vi "tcpServerSenderLoop.vi"(8 "error in (no error)":errorcluster, 10 "notifier in":refnum<notifier>, 11 "TcpServer in":refnum<class "TcpServer.lvclass">) -> (0 "error out":errorcluster, 3 "TcpServer out":refnum<class "TcpServer.lvclass">)   [LabVIEW 2018, in "TcpServer.lvclass"]
doc: "Receive an ack or an event from the LabVIEW Component to be sent to TCP Client."
uses:
  TcpServer.lvclass
  TcpServer.lvclass/TcpServer.ctl
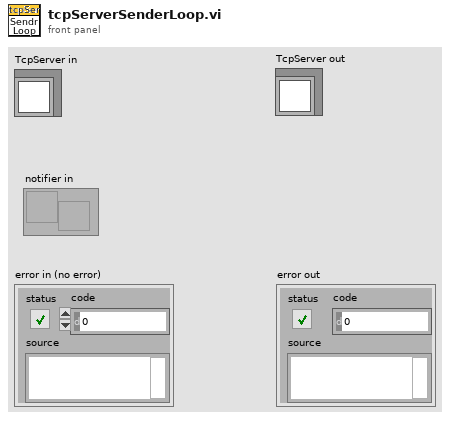
[diagram p1: front panel]
types:
  T1 = typedef "TcpServer.lvclass/packetConnIDTypeDef.ctl" = cluster{"packet":string, "firstPacket":bool, "firstConnection":bool}
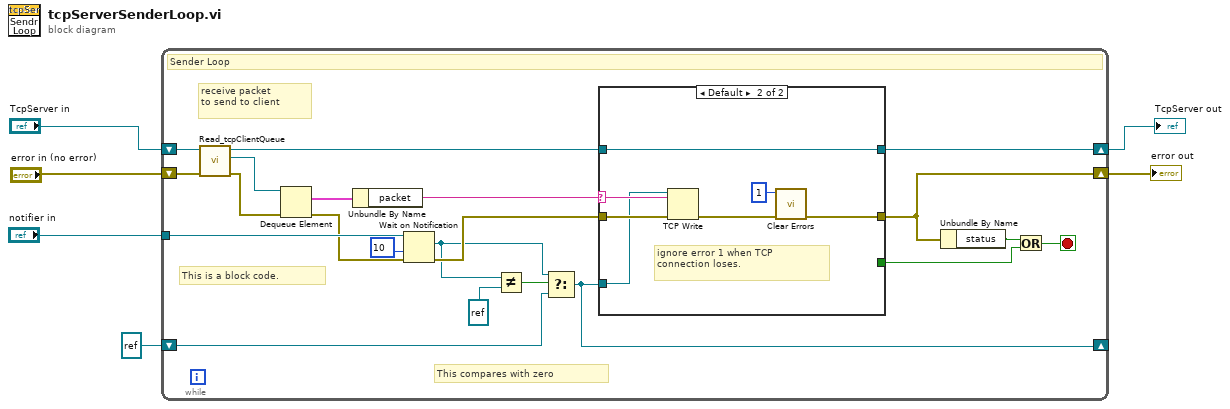
[diagram p0: block diagram]
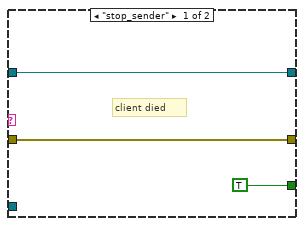
[diagram p2: hidden frame]
diagram:
  n1 = while {
    shift-right: [w21] -> w6
    shift-left: "error in (no error)" -> [w25]
    tunnel: "notifier in" -> [w17]
    shift-right: [w14] -> w2
    shift-left: "TcpServer in" -> [w27]
    shift-right: [w7] -> _
    shift-left: refnum<k5> refnum ("tcpConnectionID") -> [w8]
    stop <- w24 stop-if-true
    # "This compares with zero"
    # "This is a block code."
    # "receive packet\nto send to client"
    # "Sender Loop"
    n2 = call "Read_tcpClientQueue.vi"("error in (no error)"=w25, "tcpServer in"=w27) -> ("error out"=w18:errorcluster, "tcpClientQueue"=w26:refnum<queue>, "tcpServer out"=w15:refnum<class "TcpServer.lvclass">)  [unwired: 7 in]
    n3 = Dequeue Element(queue=w26, error in (no error)=w18) -> (element=w20:T1, error out=w12:errorcluster)  [unwired: 1 in, 2 out]
    n4 = Unbundle By Name(w20) -> ("packet"=w19:string)
    n5 = Wait on Notification(notifier=w17, timeout in ms (-1)=10, error in (no error)=w12) -> (notification=w9:refnum<k5>, error out=w11:errorcluster)  [unwired: 1 in, 2 out]
    n6 = Not Equal?(x=w9, y=refnum<k5> refnum ("tcpConnectionID")) -> (x != y?=w10:bool)
    n7 = Select(t=w9, s=w10, f=w8) -> (s? t:f=w7:refnum<k5>)
    n8 = case shown="Default" w19 {
      selector: w19 -> [_ w34]
      tunnel: [TRUE _] -> w23
      tunnel: [w28 w35] -> w21
      tunnel: w15 -> [w29 w33]
      tunnel: [w29 w33] -> w14
      tunnel: w11 -> [w28 w32]
      tunnel: w7 -> [_ w31]
      frame "stop_sender" {
        # "client died"
      }
      frame Default {
        # "ignore error 1 when TCP\nconnection loses."
        n9 = TCP Write(connection ID=w31, data in=w34, error in (no error)=w32) -> (error out=w36:errorcluster)  [unwired: 1 in, 2 out]
        n10 = call <vilib>:"Clear Errors.vi"("error in (no error)"=w36, "specific error code to clear (0: all)"=1) -> ("error out"=w35:errorcluster)  [unwired: 4 in, 1 out]
      }
    }
    n11 = Unbundle By Name(w21) -> ("status"=w22:bool)
    n12 = Or(x=w22, y=w23) -> (x .or. y?=w24:bool)
  }
  "error out" <- w6
  "TcpServer out" <- w2
